vi "Set AccessType.vi"(8 "error in":errorcluster, 10 "Value":refnum<class "Value.lvclass">, 11 "Object Type in":refnum<class "ARRAY.lvclass">) -> (0 "error out":errorcluster, 3 "Object Type out":refnum<class "ARRAY.lvclass">)   [LabVIEW 2019, in "Electronic Datasheet.lvlib" / "ARRAY.lvclass"]
uses:
  ARRAY.lvclass
  Value/Value.lvclass
  Electronic Datasheet.lvlib
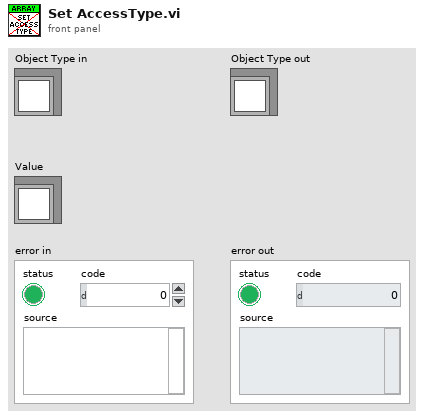
[diagram p1: front panel]
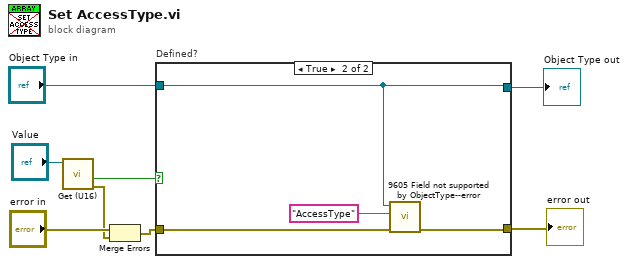
[diagram p0: block diagram]
diagram:
  n1 = call "Get (U16).vi"("Value in"="Value") -> ("error out"=w1:errorcluster, "Defined?"=w4:bool)  [unwired: 7 in, 2 out]
  n2 = Merge Errors("error in", w1) -> (w2:errorcluster)
  n3 = case "Defined?" shown="True" w4 {
    tunnel: [w10 w13] -> w6
    tunnel: "Object Type in" -> [w9 w11]
    tunnel: [w9 w11] -> w7
    tunnel: w2 -> [w10 w14]
    frame False {
    }
    frame True {
      n4 = call "9605 Field not supported by ObjectType--error.vi"("error in"=w14, "Field Name"="AccessType" ("Field name"), "Object Type Base"=w11) -> ("error out"=w13:errorcluster)  [unwired: 7 in, 1 out]
    }
  }
  "Object Type out" <- w7
  "error out" <- w6
